vi "Get Bytes.vi"(11 "MsgPackArray in":refnum<class "MsgPackArray.lvclass">) -> (2 "Array":u8[](array[numeric]), 3 "MsgPackArray out":refnum<class "MsgPackArray.lvclass">)   [LabVIEW 2020, in "MessagePack.lvlib" / "MsgPackArray.lvclass"]
uses:
  MsgPackArray.lvclass
  MsgPackArray.lvclass/MsgPackArray.ctl
  MsgPack Object Types.ctl
  MessagePack.lvclass
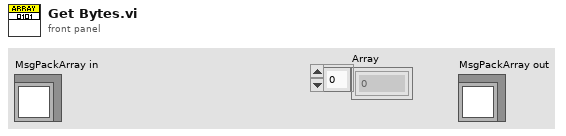
[diagram p1: front panel]
types:
  T1 = typedef "MessagePack.lvlib/MessagePack.lvclass/MsgPack Object Types.ctl" = enum16{"UNSUPPORTED", "POSINT", "NEGINT", "FIXMAP", "FIXARRAY", "FIXSTR", "NIL", "FALSE", "TRUE", "BIN8", "BIN16", "BIN32", "EXT8", "EXT16", "EXT32", "FLOAT32", "FLOAT64", "UINT8", "UINT16", "UINT32", "UINT64", "INT8", "INT16", "INT32", "INT64", "FIXEXT1", "FIXEXT2", "FIXEXT4", "FIXEXT8", "FIXEXT16", "STR8", "STR16", "STR32", "ARRAY16", "ARRAY32", "MAP16", "MAP32"}
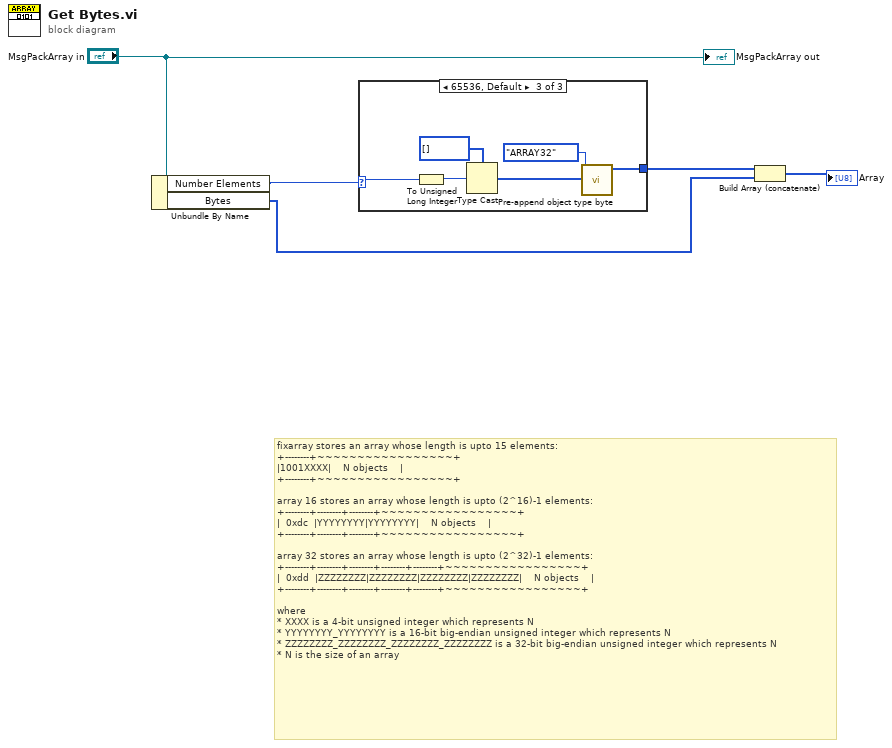
[diagram p0: block diagram]
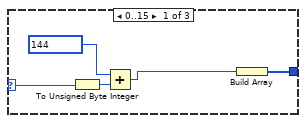
[diagram p2: hidden frame]
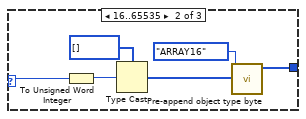
[diagram p3: hidden frame]
diagram:
  # "fixarray stores an array whose length is upto 15 elements:\n+--------+~~~~~~~~~~~~~~~~~+\n|1001XXXX|    N objects    |\n+--------+~~~~~~~~~~~~~~~~~+\n\narray 16 stores an array whose length is upto (2^16)-1 elements:\n+--------+--------+--------+~~~~~~~~~~~~~~~~~+\n|  0xdc  |YYYYYYYY|YYYYYYYY|    N objects    |\n+--------+--------+--------+~~~~~~~~~~~~~~~~~+\n\narray 32 stores an array whose length is upto (2^32)-1 elements:\n+--------+--------+--------+--------+--------+~~~~~~~~~~~~~~~~~+\n|  0xdd  |ZZZZZZZZ|ZZZZZZZZ|ZZZZZZZZ|ZZZZZZZZ|    N objects    |\n+--------+--------+--------+--------+--------+~~~~~~~~~~~~~~~~~+\n\nwhere\n* XXXX is a 4-bit unsigned integer which represents N\n* YYYYYYYY_YYYYYYYY is a 16-bit big-endian unsigned integer which represents N\n* ZZZZZZZZ_ZZZZZZZZ_ZZZZZZZZ_ZZZZZZZZ is a 32-bit big-endian unsigned integer which represents N\n* N is the size of an array"
  n1 = Unbundle By Name("MsgPackArray in") -> ("Number Elements"=w2:u32, "Bytes"=w1:u8[])
  n2 = case shown="65536, Default" w2 {
    selector: w2 -> [w9 w16 w22]
    tunnel: [w7 w12 w18] -> w4
    frame 0..15 {
      n3 = To Unsigned Byte Integer(number=w9) -> (unsigned 8bit integer=w8:u8)
      n4 = Add(x=u8 144 ("y"), y=w8) -> (x+y=w6:u8)
      n5 = Build Array(w6) -> (w7:u8[])
    }
    frame 16..65535 {
      n6 = To Unsigned Word Integer(number=w16) -> (unsigned 16bit integer=w14:u16)
      n7 = Type Cast(type=u8[] [] ("bytes"), x=w14) -> (*(type *) &x=w13:u8[])
      n8 = call "Pre-append object type byte.vi"("bytes in"=w13, "Object type"=MsgPack_Object_Types."ARRAY16") -> ("encoded bytes"=w12:u8[])  [unwired: 8 in, 1 out]
    }
    frame 65536, Default {
      n9 = To Unsigned Long Integer(number=w22) -> (unsigned 32bit integer=w20:u32)
      n10 = Type Cast(type=u8[] [] ("bytes"), x=w20) -> (*(type *) &x=w19:u8[])
      n11 = call "Pre-append object type byte.vi"("bytes in"=w19, "Object type"=MsgPack_Object_Types."ARRAY32") -> ("encoded bytes"=w18:u8[])  [unwired: 8 in, 1 out]
    }
  }
  n12 = Build Array (concatenate)(w4, w1) -> (→"Array":u8[])
  "MsgPackArray out" <- "MsgPackArray in"
